vi "Running Histogram.vi"(6 "reset":bool caption="Reset", 8 "bins":i32=20, 9 "max":dbl=10.0 format="%0.2f", 10 "min":dbl=-10.0 format="%0.2f", 11 "input data":dbl[](array[numeric])) -> (1 "total count":i32, 2 "x axis":dbl[](array[numeric]), 3 "histogram":dbl[](array[numeric]), 4 "out of range":cluster{"count below":i32, "count above":i32})   [LabVIEW 2018]
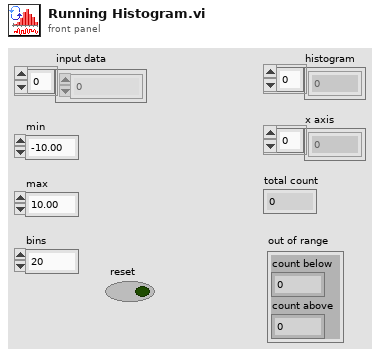
[diagram p1: front panel]
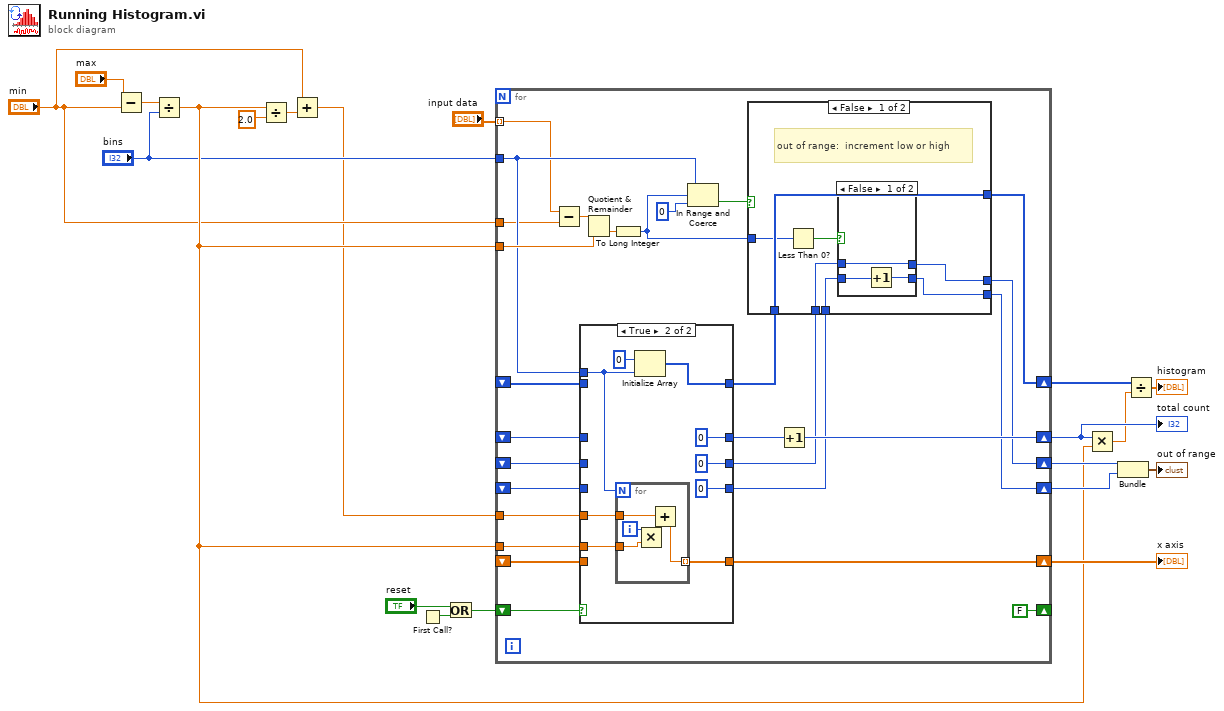
[diagram p0: block diagram]
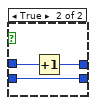
[diagram p3: hidden frame]
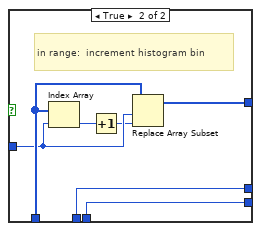
[diagram p4: hidden frame]
diagram:
  n1 = Subtract(x="max", y="min") -> (x-y=w4:dbl)
  n2 = Divide(x=w4, y="bins") -> (x/y=w7:dbl)
  n3 = Divide(x=w7, y=2.0) -> (x/y=w2:dbl)
  n4 = Add(x="min", y=w2) -> (x+y=w1:dbl)
  n5 = First Call?() -> (First Call?: T/F=w20:bool)
  n6 = Or(x="reset", y=w20) -> (x .or. y?=w18:bool)
  n7 = for {
    tunnel: "input data" -> [w40] mode=indexing
    tunnel: "min" -> [w25]
    tunnel: w7 -> [w46]
    tunnel: "bins" -> [w41]
    shift-right: [w35] -> w15
    shift-left: _ -> [w39]
    shift-right: [w29] -> w11
    shift-left: _ -> [w38]
    shift-right: [w30] -> w10
    shift-left: _ -> [w37]
    shift-right: [w27] -> w17
    shift-left: _ -> [w34]
    shift-right: [FALSE] -> _
    shift-left: w18 -> [w42]
    tunnel: w1 -> [w24]
    tunnel: w7 -> [w23]
    shift-right: [w21] -> w12
    shift-left: _ -> [w22]
    n8 = Subtract(x=w40, y=w25) -> (x-y=w47:dbl)
    n9 = case shown="True" w42 {
      tunnel: w41 -> [_ w53]
      tunnel: [w52 0 ("element")] -> w36
      tunnel: [w51 0 ("element")] -> w32
      tunnel: [w50 0 ("element")] -> w31
      tunnel: w39 -> [w52 _]
      tunnel: w38 -> [w51 _]
      tunnel: w37 -> [w50 _]
      tunnel: [w49 w57] -> w28
      tunnel: w34 -> [w49 _]
      tunnel: w24 -> [_ w56]
      tunnel: w23 -> [_ w55]
      tunnel: w22 -> [w48 _]
      tunnel: [w48 w54] -> w21
      frame False {
      }
      frame True {
        n10 = for {
          N: w53 -> [_]
          tunnel: w56 -> [w66]
          tunnel: w55 -> [w64]
          tunnel: [w62] -> w54 mode=indexing
          i -> [w65]
          n11 = Multiply(x=w65, y=w64) -> (x*y=w63:dbl)
          n12 = Add(x=w66, y=w63) -> (x+y=w62:dbl)
        }
        n13 = Initialize Array(0 ("element"), w53) -> (w57:i32[])
      }
    }
    n14 = Quotient & Remainder(x=w47, y=w46) -> (floor(x/y)=w43:dbl)  [unwired: 1 out]
    n15 = To Long Integer(number=w43) -> (32bit integer=w26:i32)
    n16 = In Range and Coerce(upper limit=w41, x=w26, lower limit=0) -> (In Range?=w44:bool)  [unwired: 1 out]
    n17 = case shown="False" w44 {
      tunnel: w32 -> [w72 w81]
      tunnel: w31 -> [w71 w80]
      tunnel: [w70 w81] -> w29
      tunnel: [w69 w80] -> w30
      tunnel: w28 -> [w68 w85]
      tunnel: [w68 w82] -> w27
      tunnel: w26 -> [w67 w84]
      frame False {
        # "out of range:  increment low or high"
        n18 = Less Than 0?(x=w67) -> (x < 0?=w73:bool)
        n19 = case shown="False" w73 {
          tunnel: w72 -> [w74 w79]
          tunnel: w71 -> [w75 w77]
          tunnel: [w74 w78] -> w70
          tunnel: [w76 w77] -> w69
          frame False {
            n20 = Increment(x=w75) -> (x+1=w76:i32)
          }
          frame True {
            n21 = Increment(x=w79) -> (x+1=w78:i32)
          }
        }
      }
      frame True {
        # "in range:  increment histogram bin"
        n22 = Index Array(array=w85, index=w84) -> (element=w86:i32)
        n23 = Increment(x=w86) -> (x+1=w83:i32)
        n24 = Replace Array Subset(array=w85, new element=w83, index=w84) -> (w82:i32[])
      }
    }
    n25 = Increment(x=w36) -> (x+1=w35:i32)
  }
  "total count" <- w15
  "x axis" <- w12
  n26 = Multiply(x=w15, y=w7) -> (x*y=w14:dbl)
  n27 = Bundle("element"=w11, "element"=w10) -> (→"out of range":cluster{"element":i32, "element":i32})  [unwired: 1 in]
  n28 = Divide(x=w17, y=w14) -> (x/y=→"histogram":dbl[])
